vi "m1m3_putSample_PowerSupplyData.vi"(8 "error in (no error)":errorcluster, 11 "PowerSupplyData_Ctl":T1) -> (0 "error out":errorcluster, 2 "function return":i32, 3 "PowerSupplyData_Ctl out":T1)   [LabVIEW 2016, in "SALLV_m1m3.lvlib"]
doc: "int m1m3_shm_putSample_PowerSupplyDataLV(m1m3_PowerSupplyDataLV *PowerSupplyData_Ctl );"
uses:
  SALLV_m1m3.lvlib
  DataTypes/PowerSupplyData.ctl
  SALLV_m1m3.so
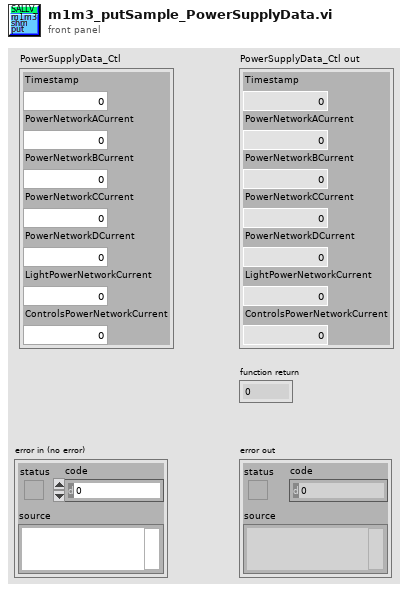
[diagram p1: front panel]
types:
  T1 = typedef "SALLV_m1m3.lvlib/PowerSupplyData.ctl" = cluster{"Timestamp":dbl, "PowerNetworkACurrent":sgl, "PowerNetworkBCurrent":sgl, "PowerNetworkCCurrent":sgl, "PowerNetworkDCurrent":sgl, "LightPowerNetworkCurrent":sgl, "ControlsPowerNetworkCurrent":sgl}
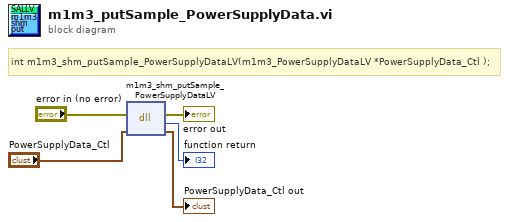
[diagram p0: block diagram]
diagram:
  # "int m1m3_shm_putSample_PowerSupplyDataLV(m1m3_PowerSupplyDataLV *PowerSupplyData_Ctl );"
  n1 = dll-call lib="opt/CODE/SALLV_m1m3/SALLV_m1m3.*" fn="m1m3_shm_putSample_PowerSupplyDataLV"(error in="error in (no error)", "PowerSupplyData_Ctl"="PowerSupplyData_Ctl") -> (error out=→"error out":errorcluster, →"function return":i32, "PowerSupplyData_Ctl"=→"PowerSupplyData_Ctl out":T1)  [unwired: 2 in, 1 out]
